vi "DFD Filtering (Wfm NChan).vi"(7 "init? (F)":bool, 8 "error in (no error)":errorcluster, 10 "filter":T1={"mSRate_Fs"=1.0, "mSRate_Version"="2.0", "mSRate_Comments"="", "mSRate_OrgCoef"={"type"=enum."Undefined", "gain"=1.0, "coef a (k)"=[], "coef b (v)"=[]}, "mSRate_CurCoef"={"type"=enum."Undefined", "gain"=1.0, "coef a (k)"=[], "coef b (v)"=[]}, "mSRate_Quantized?"=FALSE, "mSRate_QCoef"={"type"=enum."Undefined", "gain"=1.0, "coef a (k)"=[], "coef b (v)"=[]}, "mSRate_QSettings"=[], "mSRate_Order"=0, "mSRate_Scaling"={"mSRate_ScaleByPowerOf2?"=FALSE, "mSRate_ScaleType"=enum."No Norm"}} {"mSRate_QSettings"."source" items=["Coef a/k"=0, "Coef b/v"=7, "Input"=1, "Output"=2, "Multiplicand"=3, "Product"=4, "Sum"=5, "Delay"=6, "Gain"=8]}, 11 "signal in":waveform(dbl)[](array[waveform])) -> (0 "error out":errorcluster, 3 "signal out":waveform(dbl)[](array[waveform]))   [LabVIEW 2017, in "NI_DigFilterLicensed.lvlib"]
doc: "Filters an input signal continuously. Wire data to the <B>signal in</B> input to determine the polymorphic instance to use or manually select the instance."
uses:
  <vilib>/addons/Digital Filter Design/NI_DigFilterLicensed.lvlib
  <vilib>/addons/Digital Filter Design/_Objects.llb/DFD Filter Obj.ctl
  <vilib>/addons/Digital Filter Design/_Objects.llb/DFD Filter Coef.ctl
  <vilib>/addons/Digital Filter Design/_Objects.llb/DFD Filter Structure Type Selector.ctl
  <vilib>/addons/Digital Filter Design/_Objects.llb/dfd_Internal Quantization Settings.ctl
  <vilib>/addons/Digital Filter Design/_Objects.llb/dfd_Internal Quantization Srcs.ctl
  <vilib>/addons/Digital Filter Design/_Objects.llb/DFD Coef Norm Type.ctl
  <vilib>/addons/Digital Filter Design/NI_DigFilter_Process.lvlib
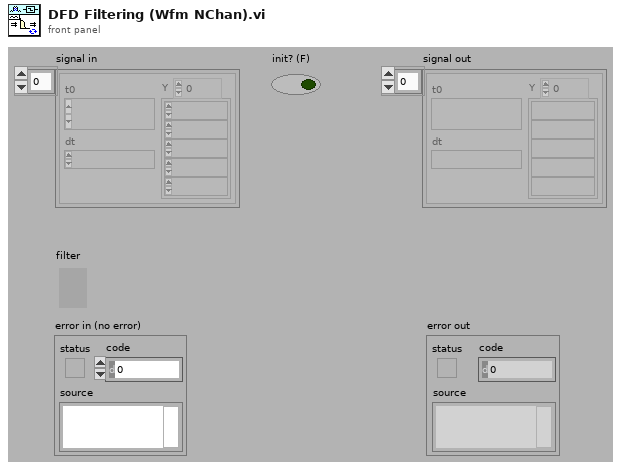
[diagram p1: front panel]
types:
  T1 = typedef "NI_DigFilterLicensed.lvlib/DFD Filter Obj.ctl" = cluster{"mSRate_Fs":dbl, "mSRate_Version":string, "mSRate_Comments":string, "mSRate_OrgCoef":T2, "mSRate_CurCoef":T2, "mSRate_Quantized?":bool, "mSRate_QCoef":T2, "mSRate_QSettings":T4[], "mSRate_Order":i32, "mSRate_Scaling":cluster{"mSRate_ScaleByPowerOf2?":bool, "mSRate_ScaleType":T6}}
  T2 = typedef "NI_DigFilterLicensed.lvlib/DFD Filter Coef.ctl" = cluster{"type":T3, "gain":dbl, "coef a (k)":dbl[], "coef b (v)":dbl[]}
  T3 = typedef "NI_DigFilterLicensed.lvlib/DFD Filter Structure Type Selector.ctl" = enum16{"Undefined", "FIR Direct Form", "FIR Direct Form Transposed", "FIR Symmetric", "FIR Antisymmetric", "IIR Direct Form I", "IIR Direct Form I Transposed", "IIR Direct Form II", "IIR Direct Form II Transposed", "IIR Cascaded Second Order Sections Form I", "IIR Cascaded Second Order Sections Form I Transposed", "IIR Cascaded Second Order Sections Form II", "IIR Cascaded Second Order Sections Form II Transposed", "Lattice Allpass (basic sections)", "Lattice Allpass (one multiplier sections)", "Lattice Allpass (normalized sections)", "Lattice AR (basic sections)", "Lattice AR (one multiplier sections)", "Lattice AR (normalized sections)", "Lattice MA (minimum phase)", "Lattice MA (maximum phase)", "Lattice ARMA (basic sections)", "Lattice ARMA (one multiplier sections)", "Lattice ARMA (normalized sections)"}
  T4 = typedef "NI_DigFilterLicensed.lvlib/dfd_Internal Quantization Settings.ctl" = cluster{"source":T5, "wl":i16, "iwl":i16, "overflow mode":enum16{"Saturation", "Wrap"}, "rounding mode":enum16{"Nearest", "Truncation"}, "signed?":bool}
  T5 = typedef "NI_DigFilterLicensed.lvlib/dfd_Internal Quantization Srcs.ctl" = u16
  T6 = typedef "NI_DigFilterLicensed.lvlib/DFD Coef Norm Type.ctl" = enum16{"No Norm", "Time Domain 1-Norm", "Time Domain 2-Norm", "Time Domain Inf-Norm"}
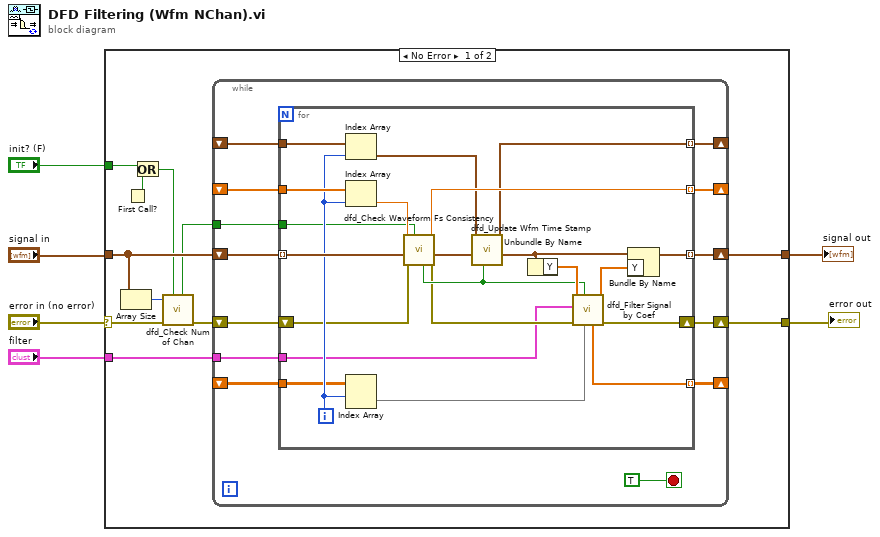
[diagram p0: block diagram]
diagram:
  n1 = case shown="No Error" "error in (no error)" {
    selector: "error in (no error)" -> [w11 w53]
    tunnel: [w7 w53] -> w3
    tunnel: "signal in" -> [w14 _]
    tunnel: [w17 _] -> w5
    tunnel: "filter" -> [w8 _]
    tunnel: "init? (F)" -> [w15 _]
    frame No Error {
      n2 = Array Size(array=w14) -> (size(s)=w13:i32)
      n3 = First Call?() -> (First Call?: T/F=w16:bool)
      n4 = Or(x=w15, y=w16) -> (x .or. y?=w12:bool)
      n5 = call <vilib>:"dfd_Check Num of Chan.vi"("init in"=w12, "error in (no error)"=w11, "#ch in"=w13) -> ("error out"=w9:errorcluster, "init out"=w10:bool)  [unwired: 7 out]
      n6 = while {
        shift-right: [w18] -> _
        shift-left: _ -> [w28]
        shift-right: [w21] -> w7
        shift-left: w9 -> [w22]
        shift-right: [w20] -> w17
        shift-left: w14 -> [w30]
        shift-right: [w26] -> _
        shift-left: _ -> [w27]
        shift-right: [w24] -> _
        shift-left: _ -> [w25]
        tunnel: w10 -> [w23]
        tunnel: w8 -> [w19]
        stop <- TRUE stop-if-true
        n7 = for {
          tunnel: w30 -> [w52] mode=indexing
          shift-right: [w38] -> w21
          shift-left: w22 -> [w42]
          tunnel: w28 -> [w32]
          tunnel: w27 -> [w51]
          tunnel: [w49] -> w26 mode=indexing
          tunnel: w25 -> [w48]
          tunnel: [w45] -> w24 mode=indexing
          tunnel: w23 -> [w43]
          tunnel: [w35] -> w20 mode=indexing
          tunnel: w19 -> [w34]
          tunnel: [w33] -> w18 mode=indexing
          i -> [w44]
          n8 = Index Array(array=w48, index=w44) -> (element=w46:timestamp)
          n9 = Index Array(array=w51, index=w44) -> (element=w50:dbl)
          n10 = Index Array(array=w32, index (row)=w44) -> (element=w31:dbl[])  [unwired: 1 in]
          n11 = call <vilib>:"dfd_Check Waveform Fs Consistency.vi"("init in"=w43, "error in (no error)"=w42, "signal in"=w52, "dt in"=w50) -> ("error out"=w39:errorcluster, "signal out"=w47:waveform(dbl), "dt out"=w49:dbl, "init out"=w40:bool)  [unwired: 4 out]
          n12 = call <vilib>:"dfd_Update Wfm Time Stamp.vi"("init? (F)"=w40, "signal in"=w47, "t0"=w46) -> ("signal out"=w37:waveform(dbl), "tf"=w45:timestamp)  [unwired: 1 in, 6 out]
          n13 = Unbundle By Name(w37) -> ("Y"=w41:dbl[])
          n14 = call <vilib>:"dfd_Filter Signal by Coef.vi"("state in"=w31, "initH?"=w40, "error in(no error)"=w39, "filter"=w34, "x"=w41) -> ("error out"=w38:errorcluster, "filtered x"=w36:dbl[], "state out"=w33:dbl[])  [unwired: 1 in, 3 out]
          n15 = Bundle By Name(cluster=w37, "Y"=w36) -> (w35:waveform(dbl))
        }
      }
    }
    frame Error {
    }
  }
  "error out" <- w3
  "signal out" <- w5
